vi "Close File.vi"(10 "File ID":string, 11 "仪器地址":u32) -> (3 "Output":string)   [LabVIEW 2010, in "DCP551.lvlib"]
uses:
  DCP551.lvlib
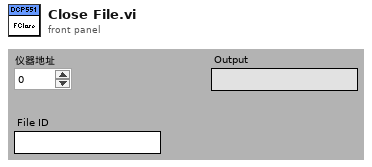
[diagram p1: front panel]
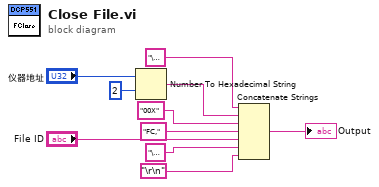
[diagram p0: block diagram]
diagram:
  n1 = Number To Hexadecimal String(1:i16 2 ("width (-)"), 2:"仪器地址") -> (0:w7:string)
  n2 = Concatenate Strings("\u0002" ("string"), w7, "00X" ("string"), "FC," ("string"), "File ID", "\u0003" ("string"), "\r\n") -> (→"Output":string)
